vi "ExFileReadNDisplayRGB.vi"() -> ()   [LabVIEW 2010]
panel:
  in  "Bit shift":u16
  in  "Type of Bayer":u32=1 max=1 step=1
  in  "Full File Name":path
  in  "?":bool
  in  "FileType":u32=67371008
  out "error out":errorcluster
  in  "error in (no error)":errorcluster
  # "File Types:\nSPE = 67371008\nTIF   = 67174400\nPMI  = 67436544"
  # "ExReadFileNDisplayRGB.vi\nThis example will read in a file of the\nselected data type and display as RGB frame.\nWhen finished viewing data, make sure to\nuse the STOP button to close the display."
  # "Browse match pattern is set to *.spe.  Modify this if different file type is needed."
  # "This will properly close\nthe image and\ndeallocate memory."
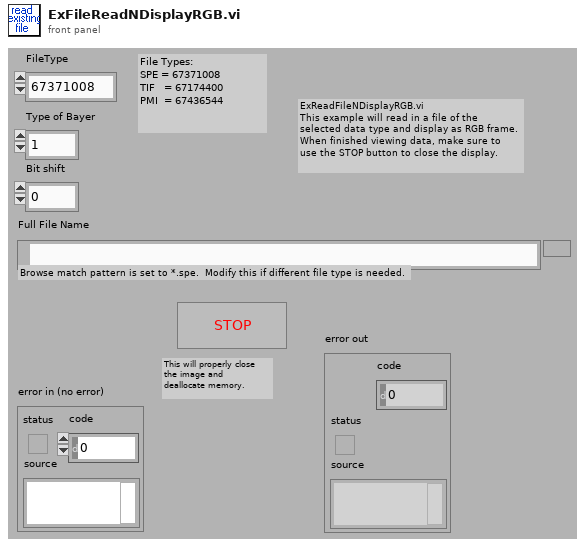
[diagram p1: front panel]
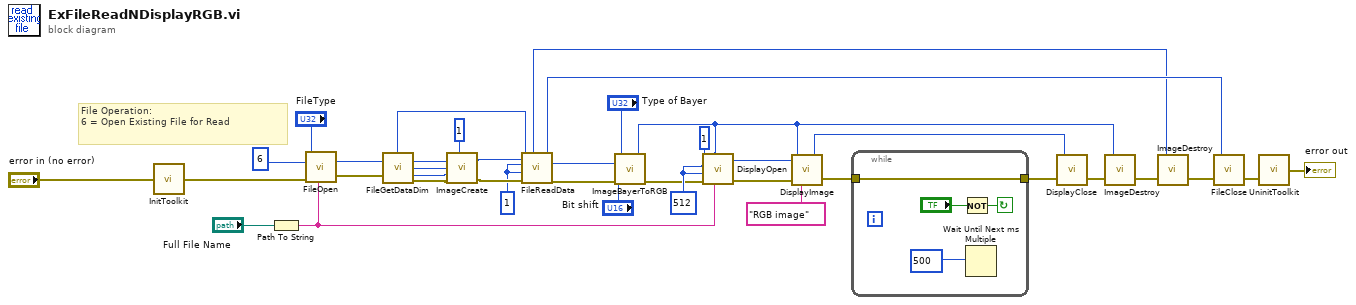
[diagram p0: block diagram]
diagram:
  w15 = 1
  w27 = 512
  # "File Operation:\n6 = Open Existing File for Read"
  n1 = call <userlib>:"InitToolkit.vi"("error in"="error in (no error)") -> ("error out"=w35:errorcluster)
  n2 = Path To String(path="Full File Name") -> (string=w21:string)
  n3 = call <userlib>:"FileOpen.vi"("error in"=w35, "File Operations"=u32 6 ("File Operation"), "FileName"=w21, "File Type"="FileType") -> ("error out"=w33:errorcluster, "File Handle"=w32:u32)
  n4 = call <userlib>:"FileGetDataDim.vi"("File Handle"=w32, "error in"=w33) -> ("Data Type"=w2:u32, "File Handle"=w18:u32, "X dim"=w30:u32, "Y dim"=w29:u32, "error out"=w31:errorcluster)  [unwired: 1 out]
  n5 = call <userlib>:"ImageCreate.vi"("X dimension"=w30, "Y dimension"=w29, "Data Type"=w2, "error in"=w31, "Number Of Frames"=1) -> ("Image Handle"=w5:u32, "error out"=w17:errorcluster)
  n6 = call <userlib>:"FileReadData.vi"("File Handle"=w18, "Start Frame"=w15, "End Frame"=w15, "error in"=w17, "Image Handle"=w5) -> ("File Handle"=w14:u32, "Image Handle"=w13:u32, "error out"=w16:errorcluster)
  n7 = call <userlib>:"ImageBayerToRGB.vi"("Image Handle"=w13, "Type of Bayer"="Type of Bayer", "Shift amount"="Bit shift", "error in"=w16) -> ("RGB Image Handle"=w6:u32, "error out"=w20:errorcluster)  [unwired: 1 in, 1 out]
  n8 = call <userlib>:"DisplayOpen.vi"("Display Title"=w21, "Image Handle"=w6, "error in"=w20, "Display Height"=w27, "Display Width"=w27, "Display Type"=1) -> ("error out"=w12:errorcluster, "Display Handle"=w11:u32)
  n9 = call <userlib>:"DisplayImage.vi"("error in"=w12, "Title"="RGB image", "Image Handle"=w6, "Display Handle"=w11) -> ("error out"=w4:errorcluster, "Display Handle"=w10:u32)
  n10 = while {
    tunnel: w4 -> [w38]
    tunnel: [w38] -> w3
    stop <- w40 continue-if-true
    n11 = Not(x="?") -> (.not. x?=w40:bool)
    n12 = Wait Until Next ms Multiple(millisecond multiple=500) -> ()  [unwired: 1 out]
  }
  n13 = call <userlib>:"DisplayClose.vi"("error in"=w3, "Display Handle"=w10) -> ("error out"=w25:errorcluster)
  n14 = call <userlib>:"ImageDestroy.vi"("error in"=w25, "Data handle"=w6) -> ("error out"=w9:errorcluster)
  n15 = call <userlib>:"ImageDestroy.vi"("error in"=w9, "Data handle"=w5) -> ("error out"=w8:errorcluster)
  n16 = call <userlib>:"FileClose.vi"("error in"=w8, "File Handle"=w14) -> ("error out"=w24:errorcluster)
  n17 = call <userlib>:"UninitToolkit.vi"("error in"=w24) -> ("error out"=→"error out":errorcluster)
